vi "EtherCAT System State Init.vi"(10 "Setup":T1, 11 "System State":map{string, dbl}(c390)) -> (3 "System State Out":map{string, dbl}(c390))   [LabVIEW 2024, in "Hardware Controller.lvlib"]
uses:
  Hardware Controller.lvlib
  EtherCAT Configuration.ctl
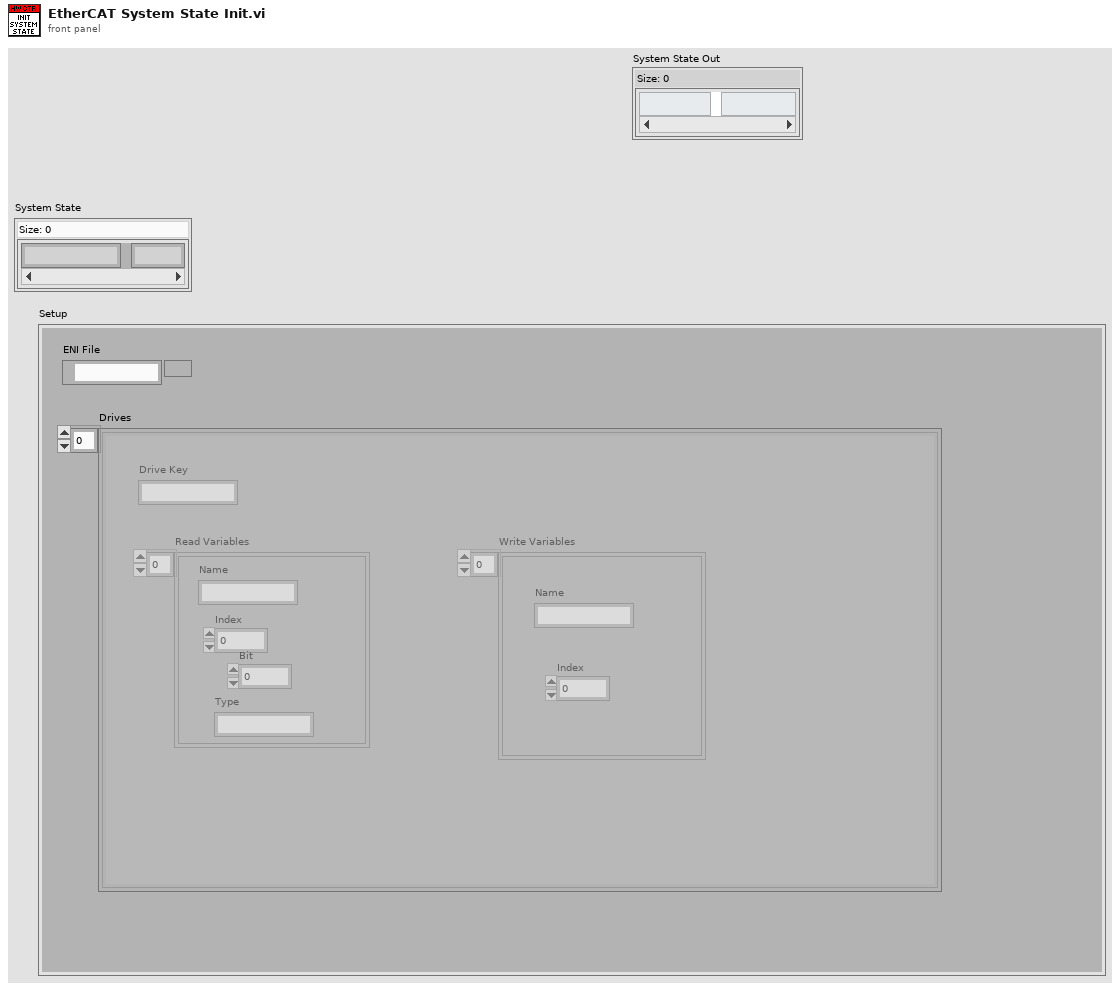
[diagram p1: front panel]
types:
  T1 = typedef "EtherCAT Configuration.ctl" = cluster{"ENI File":path, "Drives":cluster{"Drive Key":string, "Read Variables":cluster{"Name":string, "Index":u16, "Bit":u8, "Type":string}[], "Write Variables":cluster{"Name":string, "Index":u16}[]}[]}
  T2 = cluster{"Drive Key":string, "Read Variables":cluster{"Name":string, "Index":u16, "Bit":u8, "Type":string}[], "Write Variables":cluster{"Name":string, "Index":u16}[]}[]
  T3 = cluster{"Name":string, "Index":u16, "Bit":u8, "Type":string}[]
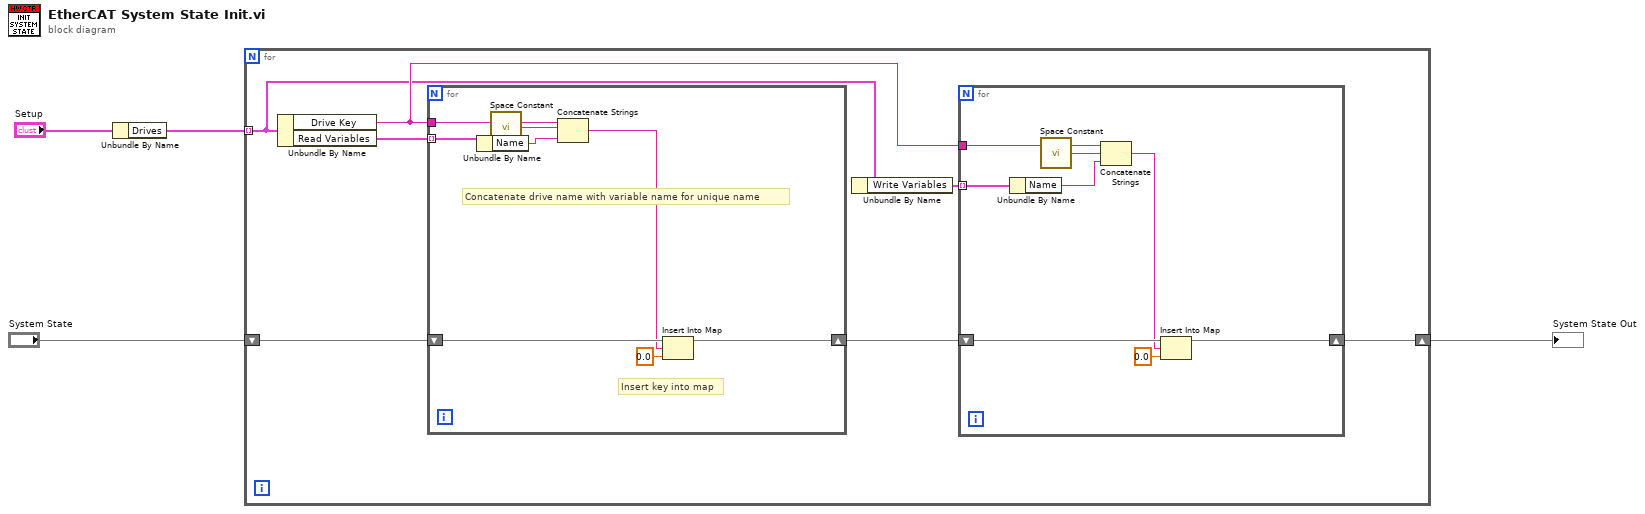
[diagram p0: block diagram]
diagram:
  n1 = Unbundle By Name("Setup") -> ("Drives"=w3:T2)
  n2 = for {
    tunnel: w3 -> [w6] mode=indexing
    shift-right: [w8] -> w1
    shift-left: "System State" -> [w10]
    n3 = Unbundle By Name(w6) -> ("Drive Key"=w7:string, "Read Variables"=w11:T3)
    n4 = for {
      tunnel: w11 -> [w25] mode=indexing
      tunnel: w7 -> [w27]
      shift-right: [w20] -> w9
      shift-left: w10 -> [w23]
      # "Insert key into map"
      # "Concatenate drive name with variable name for unique name"
      n5 = Unbundle By Name(w25) -> ("Name"=w24:string)
      n6 = call <vilib>:"Space Constant.vi"() -> ("String"=w26:string)
      n7 = Concatenate Strings(w27, w26, w24) -> (w22:string)
      n8 = Insert Into Map(map in=w23, key=w22, value=0.0) -> (map out=w20:map{string, dbl})  [unwired: 2 out]
    }
    n9 = Unbundle By Name(w6) -> ("Write Variables"=w5:cluster{"Name":string, "Index":u16}[])
    n10 = for {
      shift-right: [w14] -> w8
      shift-left: w9 -> [w15]
      tunnel: w7 -> [w19]
      tunnel: w5 -> [w16] mode=indexing
      n11 = Unbundle By Name(w16) -> ("Name"=w17:string)
      n12 = call <vilib>:"Space Constant.vi"() -> ("String"=w18:string)
      n13 = Concatenate Strings(w19, w18, w17) -> (w13:string)
      n14 = Insert Into Map(map in=w15, key=w13, value=0.0) -> (map out=w14:map{string, dbl})  [unwired: 2 out]
    }
  }
  "System State Out" <- w1
